vi "Create Pointer with Test Values.vi"(8 "error in (no error)":errorcluster) -> (0 "error out":errorcluster, 3 "Buffer out":refnum<class "Buffer.lvclass">)   [LabVIEW 2019, in "Buffer Tests.lvclass"]
uses:
  Buffer Tests.lvclass
  Classes/Buffer/Buffer.lvclass
  Classes/Buffer/Write Buffer 1D U8.vi
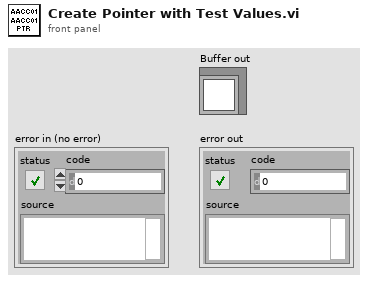
[diagram p1: front panel]
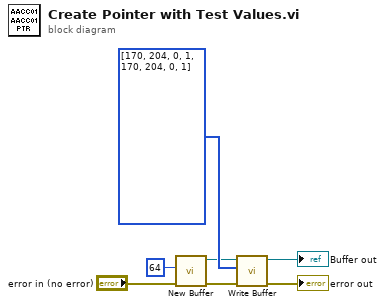
[diagram p0: block diagram]
diagram:
  n1 = call "New Buffer.vi"("error in (no error)"="error in (no error)", "buffer size"=u64 64 ("size")) -> ("error out"=w6:errorcluster, "Buffer out"=w1:refnum<class "Buffer.lvclass">)  [unwired: 8 in]
  n2 = call-poly "Write Buffer.vi"("error in (no error)"=w6, "src array in"=u8[] [170, 204, 0, 1, 170, 204, 0, 1] ("test values"), "Buffer in"=w1) -> ("error out"=→"error out":errorcluster, "Buffer out"=→"Buffer out":refnum<class "Buffer.lvclass">)  [unwired: 5 in, 2 out]
